vi "EMD8216 close.vi"(11 "CardID":u32) -> (3 "error_code":u32)   [LabVIEW 2015, in "EMD8216_64.lvlib"]
doc: "EMD8216Status EMD8216_close(u32 CardID);"
uses:
  EMD8216_64.lvlib
  EMD8216_64.dll
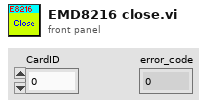
[diagram p1: front panel]
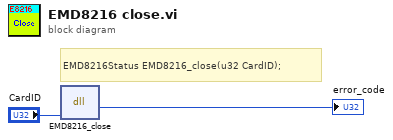
[diagram p0: block diagram]
diagram:
  # "EMD8216Status EMD8216_close(u32 CardID);"
  n1 = dll-call lib="C:/Users/jeff.lin.MINAIK/Documents/Soulkai/Labview/io/EMD8216_64/EMD8216_64/EMD8216_64.*" fn="EMD8216_close"("CardID"="CardID") -> (→"error_code":u32)  [unwired: 4 in, 2 out]
